vi "One Dynamic Input No Dynamic Output.vi"(8 "error in (no error)":errorcluster, 11 "Class Alpha in":refnum<class "Class Alpha.lvclass">) -> (0 "error out":errorcluster, 1 "Class Alpha out":refnum<class "Class Alpha.lvclass">)   [LabVIEW 2023, in "Class Alpha.lvclass"]
doc: "This VI is an example of a dynamic member VI with no dynamic output terminals. Because the class input terminal is dynamic, this VI can be override in classes that inherit from this VI's class. The class output is not a modification of the input, but rather an independent object."
uses:
  Class Alpha.lvclass
  Class Alpha.lvclass/Class Alpha.ctl
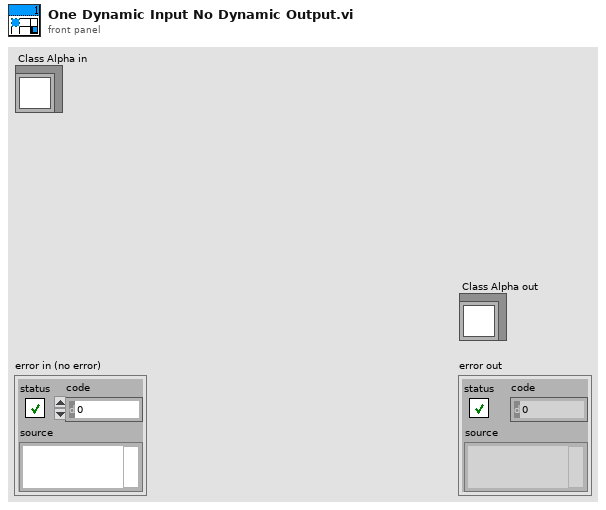
[diagram p1: front panel]
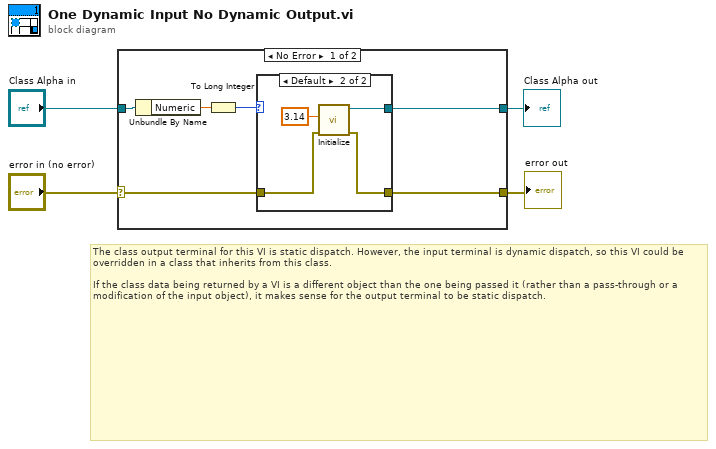
[diagram p0: block diagram]
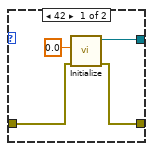
[diagram p2: hidden frame]
diagram:
  # "The class output terminal for this VI is static dispatch. However, the input terminal is dynamic dispatch, so this VI could be overridden in a class that inherits from this class.\n\nIf the class data being returned by a VI is a different object than the one being passed it (rather than a pass-through or a modification of the input object), it makes sense for the output terminal to be static dispatch."
  n1 = case shown="No Error" "error in (no error)" {
    selector: "error in (no error)" -> [w8 w20]
    tunnel: [w7 w20] -> w3
    tunnel: [w9 w19] -> w1
    tunnel: "Class Alpha in" -> [w10 w19]
    frame No Error {
      n2 = Unbundle By Name(w10) -> ("Numeric"=w6:dbl)
      n3 = To Long Integer(number=w6) -> (32bit integer=w5:i32)
      n4 = case shown="Default" w5 {
        tunnel: [w14 w18] -> w9
        tunnel: w8 -> [w13 w17]
        tunnel: [w12 w16] -> w7
        frame 42 {
          n5 = call "Initialize.vi"("error in (no error)"=w13, "Numeric"=0.0) -> ("error out"=w12:errorcluster, "Class Alpha out"=w14:refnum<class "Class Alpha.lvclass">)  [unwired: 8 in]
        }
        frame Default {
          n6 = call "Initialize.vi"("error in (no error)"=w17, "Numeric"=3.14) -> ("error out"=w16:errorcluster, "Class Alpha out"=w18:refnum<class "Class Alpha.lvclass">)  [unwired: 8 in]
        }
      }
    }
    frame Error {
    }
  }
  "error out" <- w3
  "Class Alpha out" <- w1
